vi "close.vi"(1 "error in (no error)":errorcluster) -> (0 "error out":errorcluster)   [LabVIEW 2016]
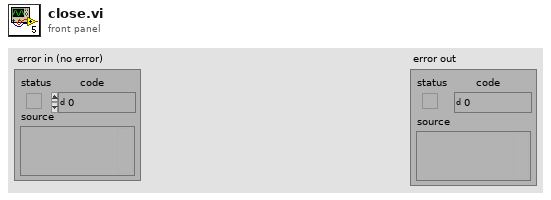
[diagram p1: front panel]
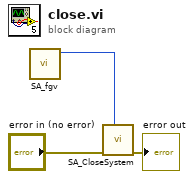
[diagram p0: block diagram]
diagram:
  n1 = call "SA_fgv.vi"() -> ("system index"=w1:u32)  [unwired: 4 in, 3 out]
  n2 = call <vilib>:"SA_CloseSystem.vi"("systemIndex"=w1, "error in (no error)"="error in (no error)") -> ("error out"=→"error out":errorcluster)  [unwired: 9 in]
